vi "Initialize.vi"(8 "error in (no error)":errorcluster, 10 "Device":string, 11 "H-Intfc in":refnum<class "REST Interface.lvclass">) -> (0 "error out":errorcluster, 3 "H-Intfc out":refnum<class "REST Interface.lvclass">)   [LabVIEW 2018, in "REST Interface.lvlib" / "REST Interface.lvclass"]
uses:
  REST Interface.lvclass
  REST Interface.lvclass/REST Interface.ctl
  PPLs/Configuration/Configuration.lvlibp/Configuration.lvclass
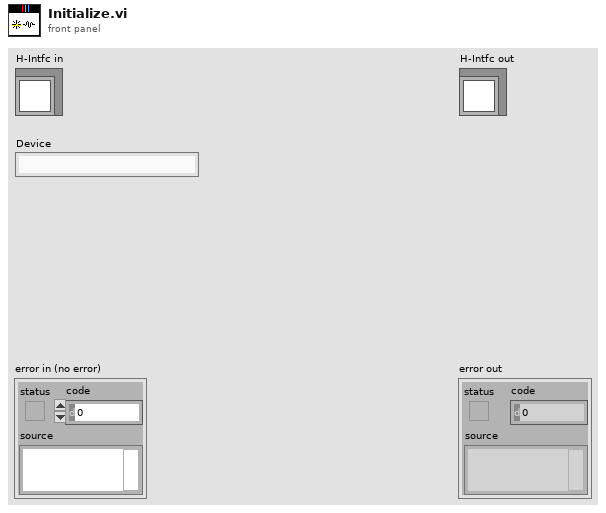
[diagram p1: front panel]
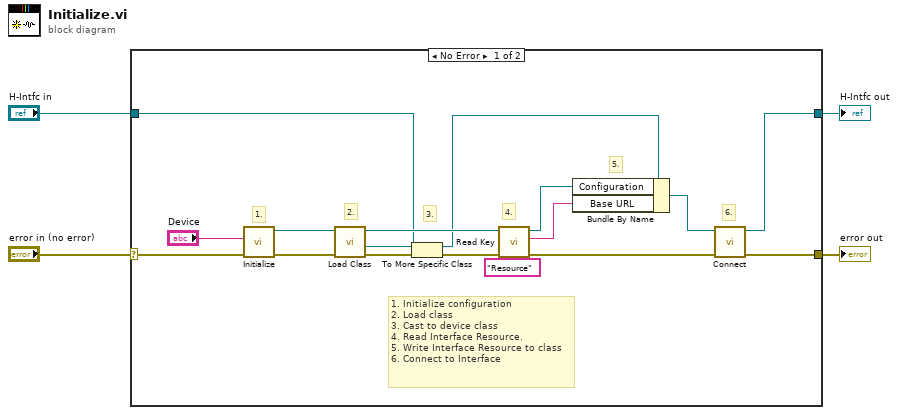
[diagram p0: block diagram]
diagram:
  n1 = case shown="No Error" "error in (no error)" {
    selector: "error in (no error)" -> [w20 w23]
    tunnel: [w9 w23] -> w3
    tunnel: [w8 w22] -> w1
    tunnel: "H-Intfc in" -> [w15 w22]
    frame No Error {
      # "5."
      # "1. Initialize configuration\n2. Load class\n3. Cast to device class\n4. Read Interface Resource.\n5. Write Interface Resource to class\n6. Connect to Interface"
      # "6."
      # "4."
      # "3."
      # "2."
      # "1."
      n2 = call "Initialize.vi"("error in"=w20, "Device"="Device") -> ("error out"=w18:errorcluster, "Configuration out"=w19:refnum<class "Configuration.lvclass">)  [unwired: 8 in]
      n3 = call "Load Class.vi"("error in"=w18, "Configuration in"=w19) -> ("error out"=w14:errorcluster, "Class out"=w17:refnum<class>, "Configuration out"=w16:refnum<class "Configuration.lvclass">)  [unwired: 7 in]
      n4 = To More Specific Class(target class=w15, reference=w17, error in=w14) -> (specific class reference=w12:refnum<class "REST Interface.lvclass">, error out=w13:errorcluster)
      n5 = call "Read Key.vi"("Key:"="Resource", "error in"=w13, "Configuration in"=w16) -> ("error out"=w6:errorcluster, "Value"=w7:string, "Configuration out"=w10:refnum<class "Configuration.lvclass">)  [unwired: 6 in]
      n6 = Bundle By Name(cluster=w12, "Configuration"=w10, "Base URL"=w7) -> (w5:refnum<class "REST Interface.lvclass">)
      n7 = call-dynamic "Connect.vi"("error in (no error)"=w6, "REST Interface in"=w5) -> ("error out"=w9:errorcluster, "REST Interface out"=w8:refnum<class "REST Interface.lvclass">)  [unwired: 8 in]
    }
    frame Error {
    }
  }
  "error out" <- w3
  "H-Intfc out" <- w1
